vi "Dataflow Tick Count ms.vi"(9 "error in":errorcluster) -> (1 "error out":errorcluster, 2 "millisecond timer value":u32)   [LabVIEW 2024, in "Common Helpers.lvlib"]
uses:
  Common Helpers.lvlib
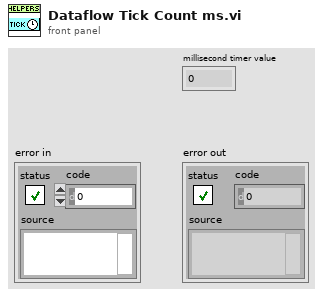
[diagram p1: front panel]
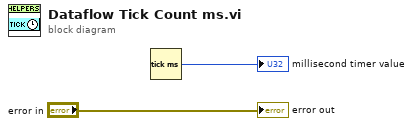
[diagram p0: block diagram]
diagram:
  n1 = Tick Count (ms)() -> (millisecond timer value=→"millisecond timer value":u32)
  "error out" <- "error in"
